vi "缺试剂配置.vi"() -> ()   [LabVIEW 2016, in "斯坦道CODMn新电路板.lvlib"]
panel:
  out "评价结果 8":u16
  out "评价结果 7":u16
  out "评价结果 6":u16
  out "评价结果 5":u16
  out "评价结果 4":u16
  out "评价结果 3":u16
  out "评价结果 2":u16
  out "评价结果":u16
  out "当前光值 8":u16
  out "当前光值 7":u16
  out "当前光值 6":u16
  out "当前光值 5":u16
  out "当前光值 4":u16
  out "当前光值 3":u16
  out "当前光值 2":u16
  out "当前光值":u16
  in  "保存":bool
  in  "数值 8":u16
  in  "数值 7":u16
  in  "数值 6":u16
  in  "数值 5":u16
  in  "数值 4":u16
  in  "数值 3":u16
  in  "数值 2":u16
  in  "数值":u16
  in  "预留(CH8):":enum8{"常量型", "通过型"}(ring)
  in  "预留(CH7):":enum8{"常量型", "通过型"}(ring)
  in  "纯水(CH6):":enum8{"常量型", "通过型"}(ring)
  in  "硫酸(CH5):":enum8{"常量型", "通过型"}(ring)
  in  "草酸钠(CH4):":enum8{"常量型", "通过型"}(ring)
  in  "高锰酸钾(CH3):":enum8{"常量型", "通过型"}(ring)
  in  "排液(CH2):":enum8{"常量型", "通过型"}(ring)
  in  "水样(CH1):":enum8{"常量型", "通过型"}(ring)
  # "当前光值(mV)"
  # "评价结果"
  # "类型选择"
  # "设置值"
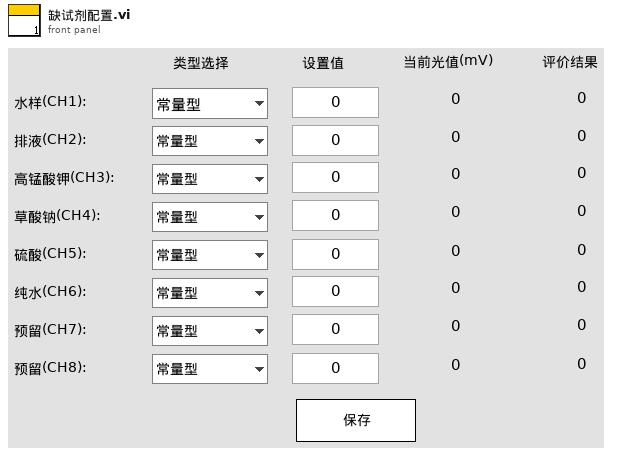
[diagram p1: front panel]
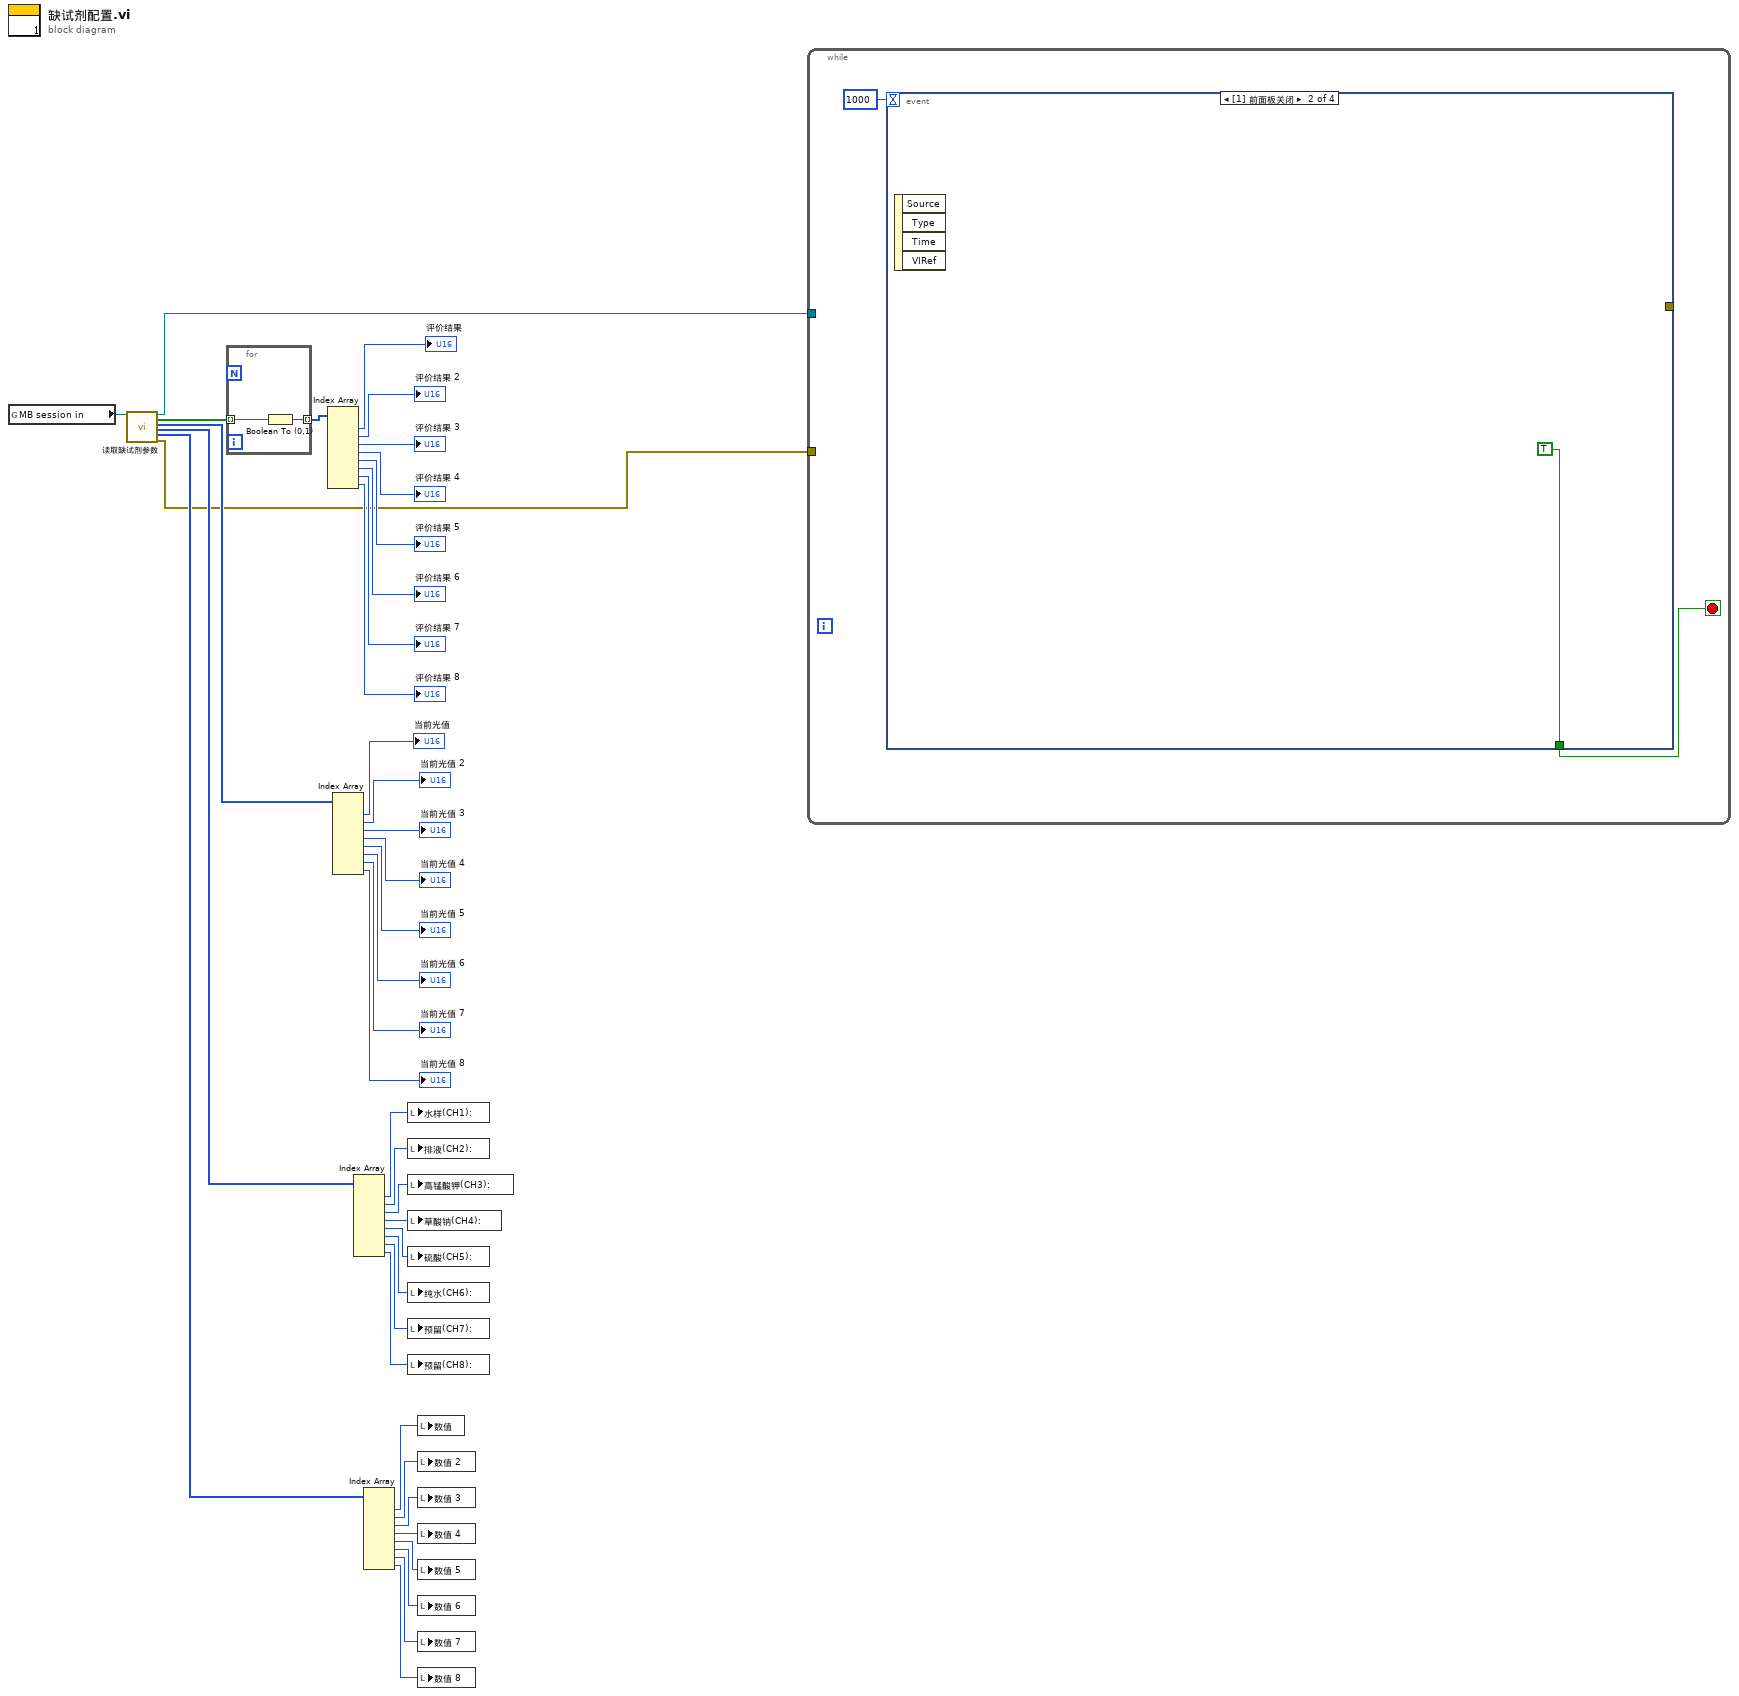
[diagram p0: block diagram]
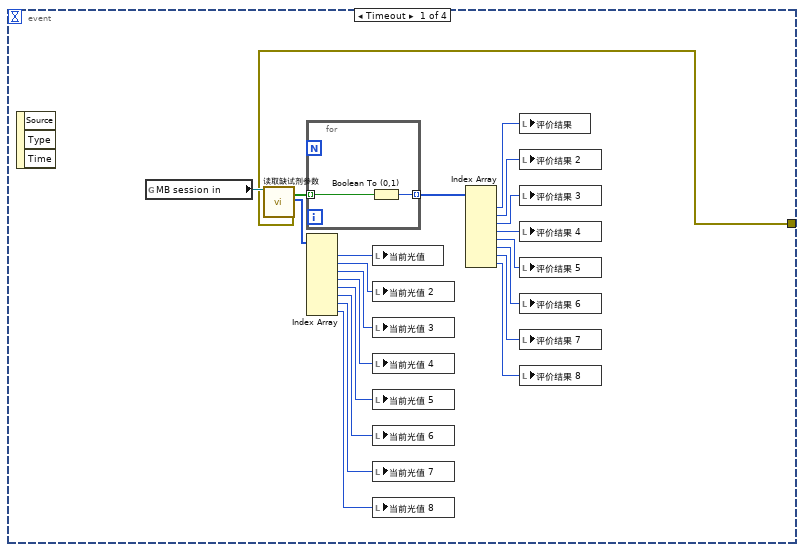
[diagram p2: hidden frame]
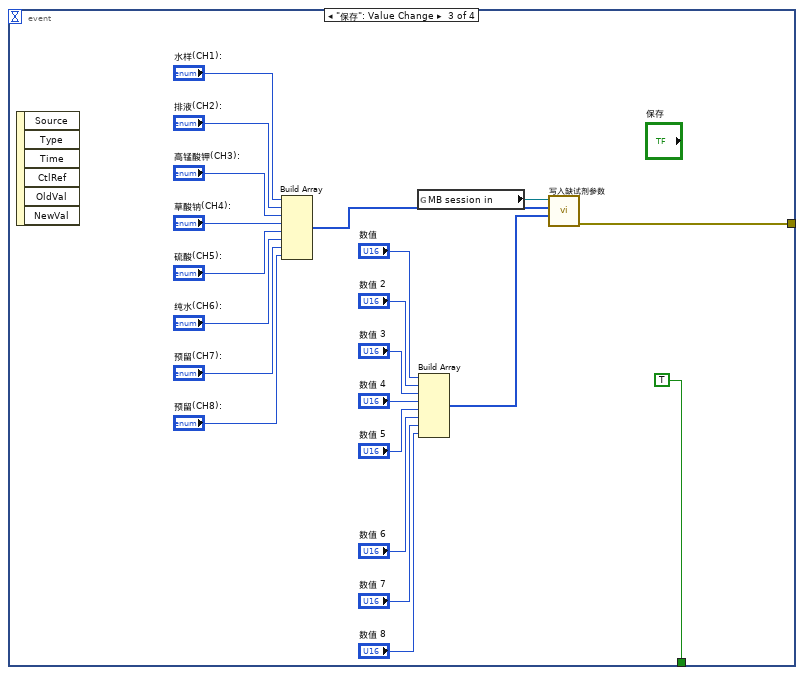
[diagram p3: hidden frame]
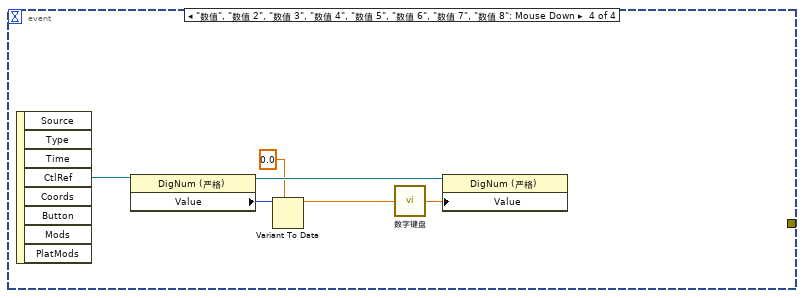
[diagram p4: hidden frame]
diagram:
  n1 = global read "VARCODMn全局变量.vi" "MB session in"() -> (w40:refnum<class "MB_Master.lvclass">)
  n2 = call "读取缺试剂参数.vi"("MB session in"=w40) -> ("MB session out"=w20:refnum<class "MB_Master.lvclass">, "评价结果"=w38:bool[], "CH光值"=w39:u16[], "缺试剂类型"=w19:u8[], "光强阈值"=w10:u16[], "error out"=w9:errorcluster)  [unwired: 13 in]
  n3 = for {
    tunnel: w38 -> [w42] mode=indexing
    tunnel: [w41] -> w37 mode=indexing
    n4 = Boolean To (0,1)(Boolean=w42) -> (0, 1=w41:i16)
  }
  n5 = Index Array(array=w37) -> (element #1=→"评价结果":i16, element #2=→"评价结果 2":i16, element #3=→"评价结果 3":i16, element #4=→"评价结果 4":i16, element #5=→"评价结果 5":i16, element #6=→"评价结果 6":i16, element #7=→"评价结果 7":i16, element #8=→"评价结果 8":i16)  [unwired: 8 in]
  n6 = Index Array(array=w39) -> (element #1=→"当前光值":u16, element #2=→"当前光值 2":u16, element #3=→"当前光值 3":u16, element #4=→"当前光值 4":u16, element #5=→"当前光值 5":u16, element #6=→"当前光值 6":u16, element #7=→"当前光值 7":u16, element #8=→"当前光值 8":u16)  [unwired: 8 in]
  n7 = Index Array(array=w19) -> (element #1=w18:u8, element #2=w17:u8, element #3=w16:u8, element #4=w15:u8, element #5=w14:u8, element #6=w13:u8, element #7=w12:u8, element #8=w11:u8)  [unwired: 8 in]
  n8 = Index Array(array=w10) -> (element #1=w8:u16, element #2=w7:u16, element #3=w6:u16, element #4=w5:u16, element #5=w4:u16, element #6=w3:u16, element #7=w2:u16, element #8=w1:u16)  [unwired: 8 in]
  n9 = local write "水样(CH1):"(w18) -> ()
  n10 = local write "排液(CH2):"(w17) -> ()
  n11 = local write "高锰酸钾(CH3):"(w16) -> ()
  n12 = local write "草酸钠(CH4):"(w15) -> ()
  n13 = local write "硫酸(CH5):"(w14) -> ()
  n14 = local write "纯水(CH6):"(w13) -> ()
  n15 = local write "预留(CH7):"(w12) -> ()
  n16 = local write "预留(CH8):"(w11) -> ()
  n17 = local write "数值"(w8) -> ()
  n18 = local write "数值 2"(w7) -> ()
  n19 = local write "数值 3"(w6) -> ()
  n20 = local write "数值 4"(w5) -> ()
  n21 = local write "数值 5"(w4) -> ()
  n22 = local write "数值 6"(w3) -> ()
  n23 = local write "数值 7"(w2) -> ()
  n24 = local write "数值 8"(w1) -> ()
  n25 = while {
    tunnel: w20 -> [_]
    tunnel: w9 -> [_]
    stop <- w44 stop-if-true
    n26 = event shown="[1] 前面板关闭" {
      selector: _ -> [_ _ _ _]
      dyn-events: _ -> [_ _ _ _]
      timeout: 1000 -> [_ _ _ _]
      tunnel: [_ TRUE TRUE _] -> w44
      tunnel: [w64 _ w87 _] -> _
      event Timeout {
        n27 = event-data() -> ()  [unwired: 1 in, 3 out]
        n28 = global read "VARCODMn全局变量.vi" "MB session in"() -> (w65:refnum<class "MB_Master.lvclass">)
        n29 = call "读取缺试剂参数.vi"("MB session in"=w65) -> ("评价结果"=w63:bool[], "CH光值"=w53:u16[], "error out"=w64:errorcluster)  [unwired: 13 in, 3 out]
        n30 = for {
          tunnel: w63 -> [w67] mode=indexing
          tunnel: [w66] -> w62 mode=indexing
          n31 = Boolean To (0,1)(Boolean=w67) -> (0, 1=w66:i16)
        }
        n32 = Index Array(array=w53) -> (element #1=w52:u16, element #2=w51:u16, element #3=w50:u16, element #4=w49:u16, element #5=w48:u16, element #6=w47:u16, element #7=w46:u16, element #8=w45:u16)  [unwired: 8 in]
        n33 = local write "当前光值"(w52) -> ()
        n34 = local write "当前光值 2"(w51) -> ()
        n35 = local write "当前光值 3"(w50) -> ()
        n36 = local write "当前光值 4"(w49) -> ()
        n37 = local write "当前光值 5"(w48) -> ()
        n38 = local write "当前光值 6"(w47) -> ()
        n39 = local write "当前光值 7"(w46) -> ()
        n40 = local write "当前光值 8"(w45) -> ()
        n41 = Index Array(array=w62) -> (element #1=w61:i16, element #2=w60:i16, element #3=w59:i16, element #4=w58:i16, element #5=w57:i16, element #6=w56:i16, element #7=w55:i16, element #8=w54:i16)  [unwired: 8 in]
        n42 = local write "评价结果"(w61) -> ()
        n43 = local write "评价结果 2"(w60) -> ()
        n44 = local write "评价结果 3"(w59) -> ()
        n45 = local write "评价结果 4"(w58) -> ()
        n46 = local write "评价结果 5"(w57) -> ()
        n47 = local write "评价结果 6"(w56) -> ()
        n48 = local write "评价结果 7"(w55) -> ()
        n49 = local write "评价结果 8"(w54) -> ()
      }
      event Panel Close {
        n50 = event-data() -> ()  [unwired: 1 in, 4 out]
      }
      event "保存": Value Change {
        n51 = event-data() -> ()  [unwired: 1 in, 6 out]
        n52 = Build Array("水样(CH1):", "排液(CH2):", "高锰酸钾(CH3):", "草酸钠(CH4):", "硫酸(CH5):", "纯水(CH6):", "预留(CH7):", "预留(CH8):") -> (w78:enum8{"常量型", "通过型"}[])
        n53 = global read "VARCODMn全局变量.vi" "MB session in"() -> (w88:refnum<class "MB_Master.lvclass">)
        n54 = Build Array("数值", "数值 2", "数值 3", "数值 4", "数值 5", "数值 6", "数值 7", "数值 8") -> (w69:u16[])
        n55 = call "写入缺试剂参数.vi"("光强阈值"=w69, "缺试剂类型"=w78, "MB session in"=w88) -> ("error out"=w87:errorcluster)  [unwired: 7 in, 1 out]
      }
      event "数值", "数值 2", "数值 3", "数值 4", "数值 5", "数值 6", "数值 7", "数值 8": Mouse Down {
        n56 = event-data() -> ("CtlRef"=w90:refnum<vi>)  [unwired: 1 in, 7 out]
        n57 = property class="DigNum (严格)"(reference=w90) -> (reference out=w95:refnum<vi>, "Value"=w93:u16)  [unwired: 1 in, 1 out]
        n58 = Variant To Data(type=0.0 ("OldNumber"), Variant=w93) -> (data=w91:dbl)  [unwired: 1 in, 1 out]
        n59 = call "数字键盘.vi"("OldNumber"=w91) -> ("NewNumber"=w94:dbl)
        n60 = property class="DigNum (严格)"(reference=w95, "Value"=w94) -> ()  [unwired: 1 in, 2 out]
      }
    }
  }
